vi "DB read & write data type.vi"(6 "read/write":u16(ring) items=["Read", "Write"], 10 "database cluster write data in":T1, 11 "database cluster read data in":T1) -> (2 "database cluster write out":T1, 3 "database cluster out":T1)   [LabVIEW 2015]
uses:
  database cluster.ctl
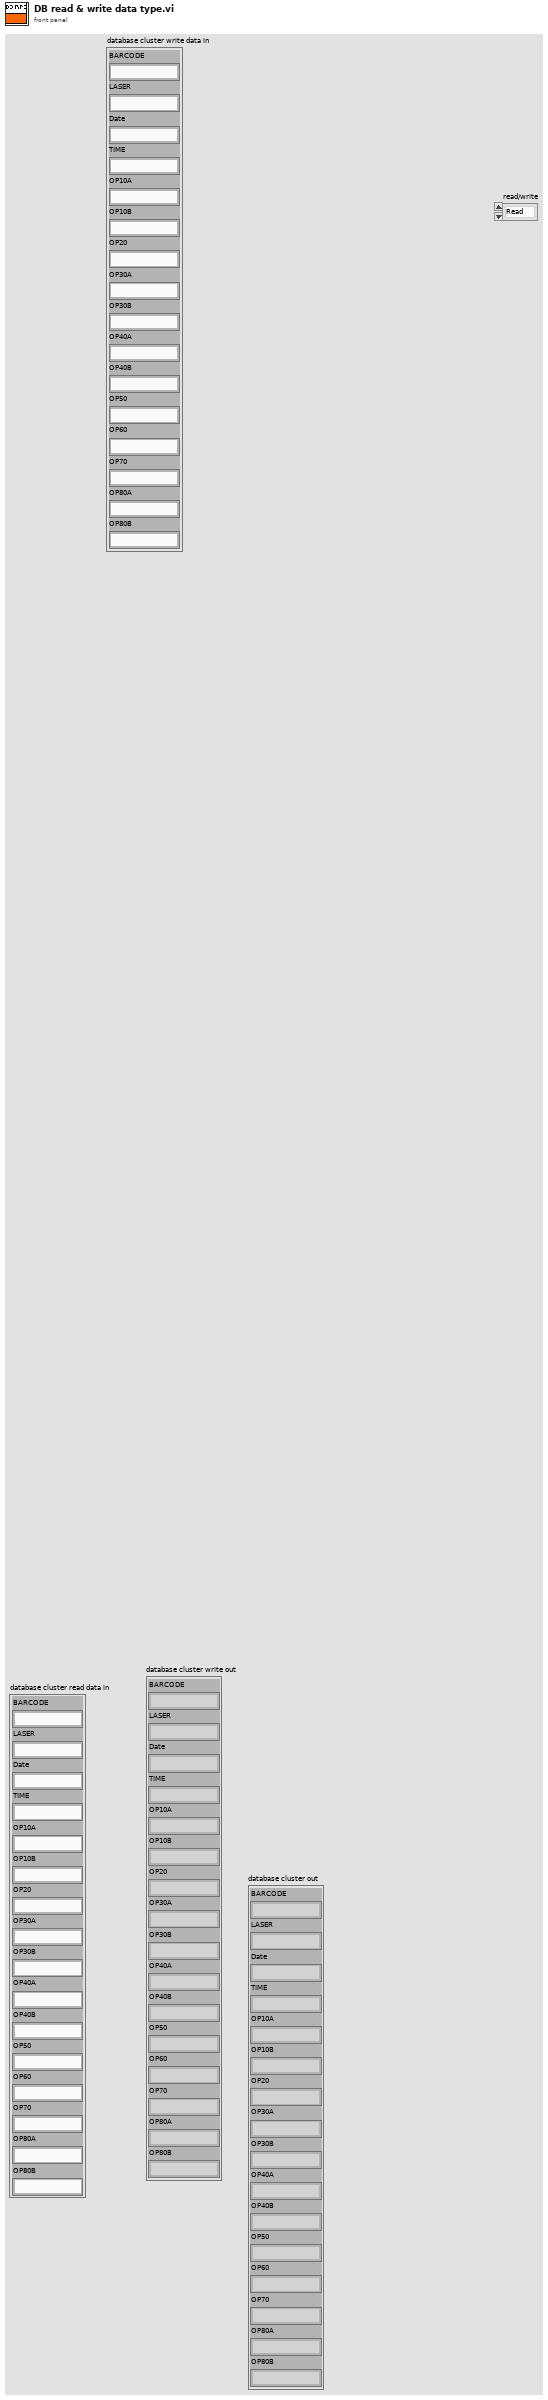
[diagram p1: front panel]
types:
  T1 = typedef "database cluster.ctl" = cluster{"BARCODE":string, "LASER":string, "Date":string, "TIME":string, "OP10A":string, "OP10B":string, "OP20":string, "OP30A":string, "OP30B":string, "OP40A":string, "OP40B":string, "OP50":string, "OP60":string, "OP70":string, "OP80A":string, "OP80B":string}
  T2 = cluster{"Company Name":string, "Model Name":string, "Part No":string, "Identify No":string, "LED1":bool, "LED1":string, "LED2":bool, "LED2":string, "LED3":bool, "LED3":string, "LED4":bool, "LED4":string, "LED5":bool, "LED5":string, "LED6":bool, "LED6":string, "LED7":bool, "LED7":string, "LED8":bool, "LED8":string, "SC1":bool, "SC1 Min":dbl, "SC1 Max":dbl, "SC2":bool, "SC2 Min ":dbl, "SC2 Max":dbl, "SC3":bool, "SC3 Min":dbl, "SC3 Max":dbl, "SC4":bool, "SC4 Min":dbl, "SC4 Max":dbl, "mv SC1":bool, "SC1 mv Min":dbl, "SC1 mv Max":dbl, "mv SC2":bool, "SC2 mv Min":dbl, "SC2 mv Max ":dbl, "mv SC3":bool, "SC3 mv Min":dbl, "SC3 mv Max":dbl, "mv SC4":bool, "SC4 mv Min":dbl, "SC4 mv Max":dbl, "MT":bool, "MotorTemp Min":dbl, "MotorTemp Max":dbl, "Temp":bool, "Temp Min":dbl, "Temp Max":dbl, "Volt":bool, "Volt.  Min":dbl, "Volt. Max":dbl, "Force":bool, "Force Min":dbl, "Force Max":dbl, "Force 2":bool, "Tr.Angle Min":dbl, "Tr.Angle Max":dbl}
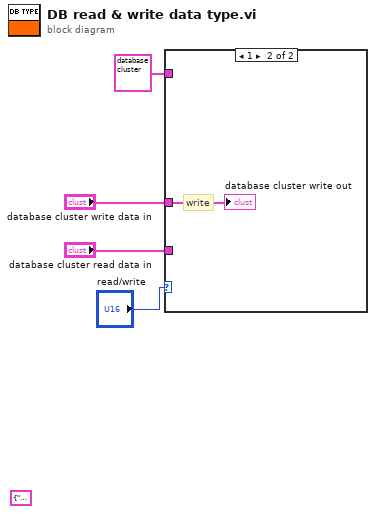
[diagram p0: block diagram]
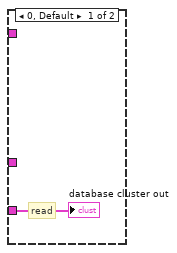
[diagram p2: hidden frame]
diagram:
  (unwired) T2 {"Company Name"="", "Model Name"="", "Part No"="", "Identify No"="", "LED1"=FALSE, "LED1"="", "LED2"=FALSE, "LED2"="", "LED3"=FALSE, "LED3"="", "LED4"=FALSE, "LED4"="", "LED5"=FALSE, "LED5"="", "LED6"=FALSE, "LED6"="", "LED7"=FALSE, "LED7"="", "LED8"=FALSE, "LED8"="", "SC1"=FALSE, "SC1 Min"=0.0, "SC1 Max"=0.0, "SC2"=FALSE, "SC2 Min "=0.0, "SC2 Max"=0.0, "SC3"=FALSE, "SC3 Min"=0.0, "SC3 Max"=0.0, "SC4"=FALSE, "SC4 Min"=0.0, "SC4 Max"=0.0, "mv SC1"=FALSE, "SC1 mv Min"=0.0, "SC1 mv Max"=0.0, "mv SC2"=FALSE, "SC2 mv Min"=0.0, "SC2 mv Max "=0.0, "mv SC3"=FALSE, "SC3 mv Min"=0.0, "SC3 mv Max"=0.0, "mv SC4"=FALSE, "SC4 mv Min"=0.0, "SC4 mv Max"=0.0, "MT"=FALSE, "MotorTemp Min"=0.0, "MotorTemp Max"=0.0, "Temp"=FALSE, "Temp Min"=0.0, "Temp Max"=0.0, "Volt"=FALSE, "Volt.  Min"=0.0, "Volt. Max"=0.0, "Force"=FALSE, "Force Min"=0.0, "Force Max"=0.0, "Force 2"=FALSE, "Tr.Angle Min"=0.0, "Tr.Angle Max"=0.0} ("Part setup 2")
  n1 = case shown="1" "read/write" {
    tunnel: "database cluster write data in" -> [_ w6]
    tunnel: T1 {"BARCODE"="", "LASER"="", "Date"="", "TIME"="", "OP10A"="", "OP10B"="", "OP20"="", "OP30A"="", "OP30B"="", "OP40A"="", "OP40B"="", "OP50"="", "OP60"="", "OP70"="", "OP80A"="", "OP80B"=""} ("Part setup") -> [_ _]
    tunnel: "database cluster read data in" -> [w5 _]
    frame 0, Default {
      # "read"
      "database cluster out" <- w5
    }
    frame 1 {
      # "write"
      "database cluster write out" <- w6
    }
  }
